vi "Get Correct Target.vi"(0 "1":bool, 1 "2":bool, 2 "Target Info":T1(array[cluster]), 3 "3":bool, 4 "4":bool) -> (5 "Position":cluster{"X":dbl, "Y":dbl})   [LabVIEW 2011]
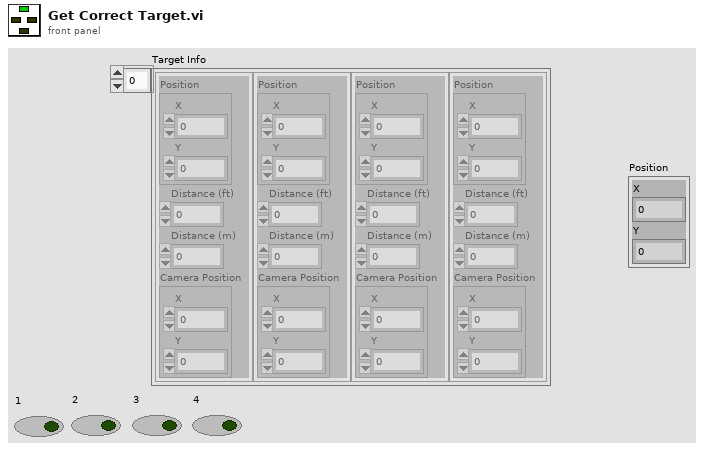
[diagram p1: front panel]
types:
  T1 = cluster{"Position":cluster{"X":dbl, "Y":dbl}, "Distance (ft)":dbl, "Distance (m)":dbl, "Camera Position":cluster{"X":dbl, "Y":dbl}}[]
  T2 = cluster{"Position":cluster{"X":dbl, "Y":dbl}, "Distance (ft)":dbl, "Distance (m)":dbl, "Camera Position":cluster{"X":dbl, "Y":dbl}}
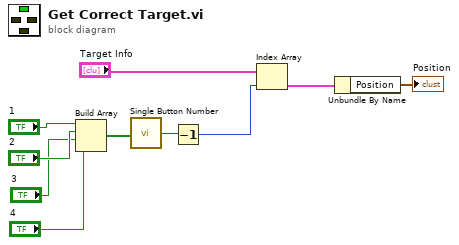
[diagram p0: block diagram]
diagram:
  n1 = Build Array("1", "2", "3", "4") -> (w6:bool[])
  n2 = call "Single Button Number.vi"("Bool Array"=w6) -> ("Number"=w5:i32)
  n3 = Decrement(x=w5) -> (x-1=w4:i32)
  n4 = Index Array(array="Target Info", index=w4) -> (element=w3:T2)
  n5 = Unbundle By Name(w3) -> ("Position"=→"Position":cluster{"X":dbl, "Y":dbl})
